vi "SysTopicInfo.vi"(8 "error in (no error)":errorcluster, 11 "MQTT1 in":refnum<class "MQTT1.lvclass">) -> (0 "error out":errorcluster, 1 "Sys Topic Descriptions":string[](array[string]), 2 "Sys Topics":string[](array[string]), 3 "MQTT1 out":refnum<class "MQTT1.lvclass">)   [LabVIEW 2017, in "MQTT1.lvclass"]
uses:
  MQTT1.lvclass
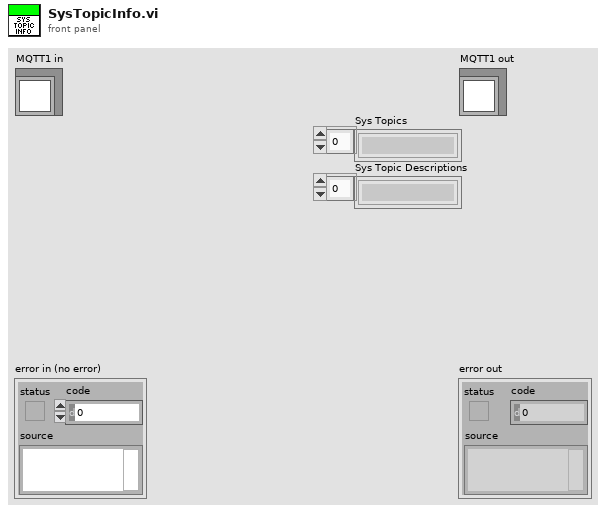
[diagram p1: front panel]
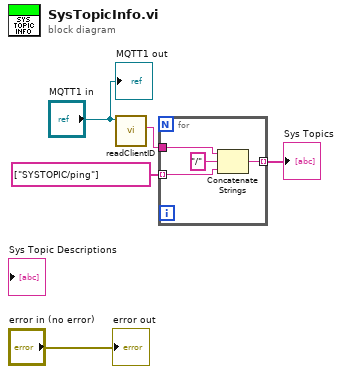
[diagram p0: block diagram]
diagram:
  n1 = call-dynamic "readClientID.vi"("MQTTclient in"="MQTT1 in") -> ("ClientId"=w2:string)  [unwired: 8 in, 2 out]
  n2 = for {
    tunnel: string[] ["SYSTOPIC/ping"] -> [w7] mode=indexing
    tunnel: w2 -> [w9]
    tunnel: [w6] -> w1 mode=indexing
    n3 = Concatenate Strings(w9, "/" ("string"), w7) -> (w6:string)
  }
  "Sys Topics" <- w1
  "error out" <- "error in (no error)"
  "MQTT1 out" <- "MQTT1 in"
